vi "Server_L.vi"(8 "stop":bool, 9 "port":u16=13078, 10 "Wait(ms)":i32=500, 11 "Server Name":string="TCPService") -> ()   [LabVIEW 2012]
panel:
  out "error out":errorcluster
  in  "error in":errorcluster
  out "Host_IP":string
  out "Users":i32 caption="#Users"
  out "Active":bool
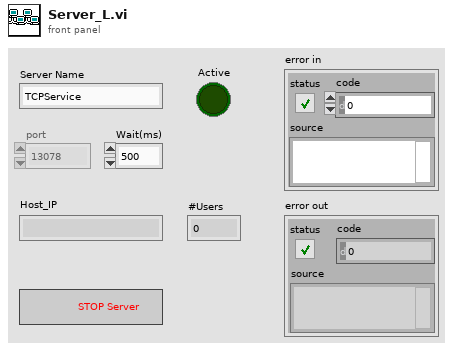
[diagram p1: front panel]
types:
  T1 = cluster{"rem addr":string, "conn ID":refnum<k5>}[]
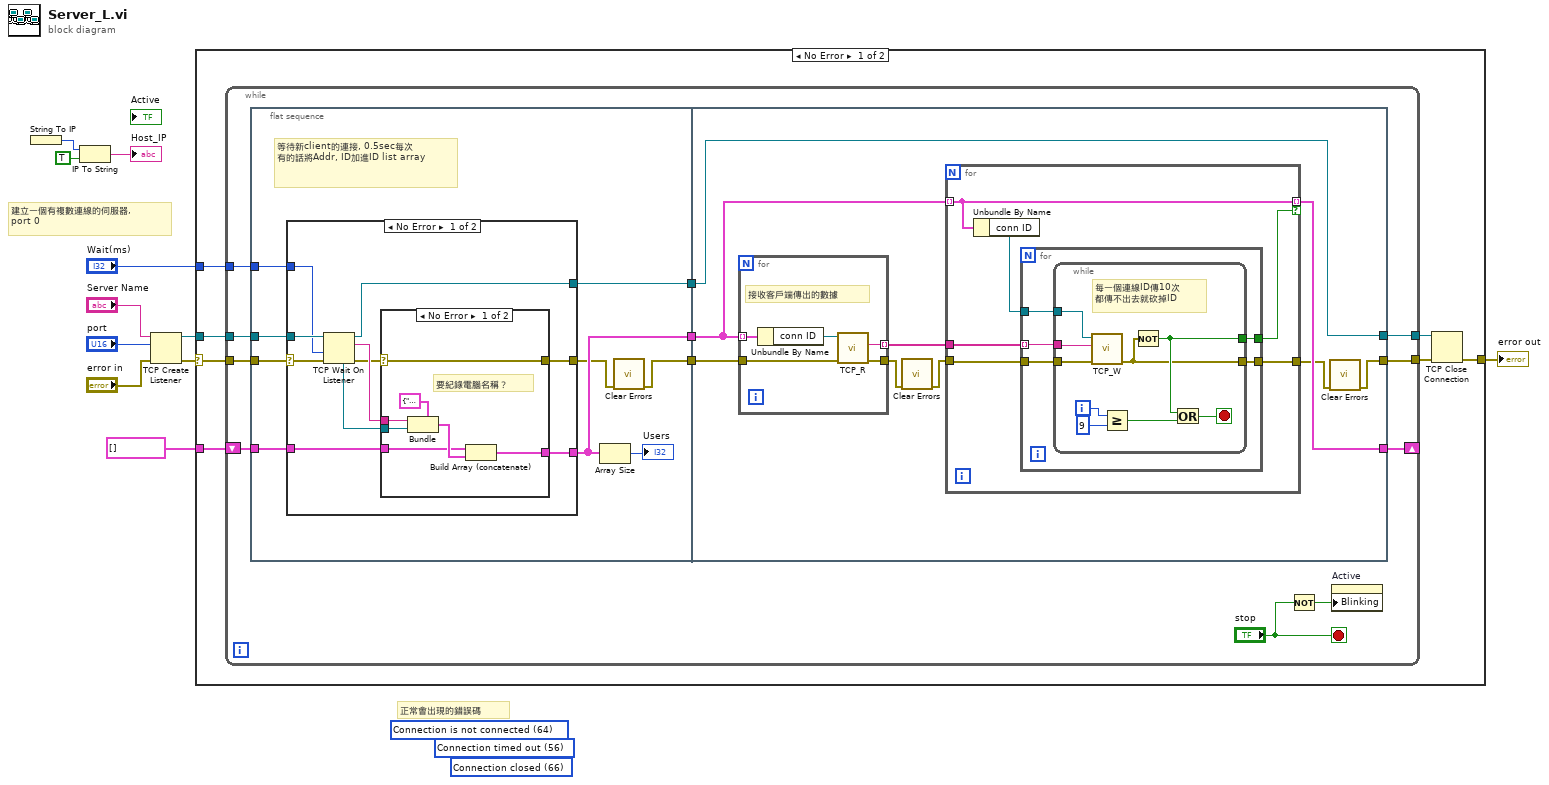
[diagram p0: block diagram]
diagram:
  (unwired) 56 items=["No Error", "Argument Error", "Memory Full", "Out of Zone", "End of File", "File Already Open", "Generic File IO Error", "File Not Found", "File Permission Error", "Disk Full", "Duplicate Path", "Too Many Files Open", "Not Enabled", "Resource File Not Found", "Cannot Add Resource", "Resource Not Found", "Image Not Found", "Image Memory Error", "Pen Does Not Exist", "Config Bad Type", "Config Token Not Found", "Config Parse Error", "Config Memory Error", "Bad External Code Format", "Bad External Code Offset", "External Code Not Present", "Null Window", "Destroy Window Mixup", "Null Menu", "Print Aborted", "Bad Print Record", "Print Driver Error", "Windows Error During Print", "Memory Error During Print", "Print Dialog Error", "Generic Print Error", "Invalid Device Refnum", "Device Not Found", "Device Parameter Error", "Device Unit Error", "Can't Open Device", "Device Call Aborted", "Generic Error", "Cancelled By User", "Object ID Too Low", "Object ID Too High", "Object Not In Heap", "Unknown Heap", "Bad DefProc ID", "DefProc Not In Table", "Message Out Of Range", "Null Method", "Unknown Message", "Manager Call Not Supported", "Bad address", "Connection In progress", "Connection timed out", "Connection is already in progress", "Network attribute not supported", "Network error", "Address in use", "System out of memory", "Connection aborted", "Connection refused", "Connection is not connected", "Connection is already connected", "Connection closed", "Initialize error (interapplication manager)", "Bad occurrence", "Wait on unbound occurrence handler", "Occurrence queue overflow", "Bad path", "Semaphore not signaled", "Unrecognized type (interapplication manager)"] ("2nd Error to Convert")
  (unwired) 66 items=["No Error", "Argument Error", "Memory Full", "Out of Zone", "End of File", "File Already Open", "Generic File IO Error", "File Not Found", "File Permission Error", "Disk Full", "Duplicate Path", "Too Many Files Open", "Not Enabled", "Resource File Not Found", "Cannot Add Resource", "Resource Not Found", "Image Not Found", "Image Memory Error", "Pen Does Not Exist", "Config Bad Type", "Config Token Not Found", "Config Parse Error", "Config Memory Error", "Bad External Code Format", "Bad External Code Offset", "External Code Not Present", "Null Window", "Destroy Window Mixup", "Null Menu", "Print Aborted", "Bad Print Record", "Print Driver Error", "Windows Error During Print", "Memory Error During Print", "Print Dialog Error", "Generic Print Error", "Invalid Device Refnum", "Device Not Found", "Device Parameter Error", "Device Unit Error", "Can't Open Device", "Device Call Aborted", "Generic Error", "Cancelled By User", "Object ID Too Low", "Object ID Too High", "Object Not In Heap", "Unknown Heap", "Bad DefProc ID", "DefProc Not In Table", "Message Out Of Range", "Null Method", "Unknown Message", "Manager Call Not Supported", "Bad address", "Connection In progress", "Connection timed out", "Connection is already in progress", "Network attribute not supported", "Network error", "Address in use", "System out of memory", "Connection aborted", "Connection refused", "Connection is not connected", "Connection is already connected", "Connection closed", "Initialize error (interapplication manager)", "Bad occurrence", "Wait on unbound occurrence handler", "Occurrence queue overflow", "Bad path", "Semaphore not signaled", "Unrecognized type (interapplication manager)"] ("3rd Error to Convert")
  (unwired) 64 items=["No Error", "Argument Error", "Memory Full", "Out of Zone", "End of File", "File Already Open", "Generic File IO Error", "File Not Found", "File Permission Error", "Disk Full", "Duplicate Path", "Too Many Files Open", "Not Enabled", "Resource File Not Found", "Cannot Add Resource", "Resource Not Found", "Image Not Found", "Image Memory Error", "Pen Does Not Exist", "Config Bad Type", "Config Token Not Found", "Config Parse Error", "Config Memory Error", "Bad External Code Format", "Bad External Code Offset", "External Code Not Present", "Null Window", "Destroy Window Mixup", "Null Menu", "Print Aborted", "Bad Print Record", "Print Driver Error", "Windows Error During Print", "Memory Error During Print", "Print Dialog Error", "Generic Print Error", "Invalid Device Refnum", "Device Not Found", "Device Parameter Error", "Device Unit Error", "Can't Open Device", "Device Call Aborted", "Generic Error", "Cancelled By User", "Object ID Too Low", "Object ID Too High", "Object Not In Heap", "Unknown Heap", "Bad DefProc ID", "DefProc Not In Table", "Message Out Of Range", "Null Method", "Unknown Message", "Manager Call Not Supported", "Bad address", "Connection In progress", "Connection timed out", "Connection is already in progress", "Network attribute not supported", "Network error", "Address in use", "System out of memory", "Connection aborted", "Connection refused", "Connection is not connected", "Connection is already connected", "Connection closed", "Initialize error (interapplication manager)", "Bad occurrence", "Wait on unbound occurrence handler", "Occurrence queue overflow", "Bad path", "Semaphore not signaled", "Unrecognized type (interapplication manager)"] ("1st Error to Convert")
  # "正常會出現的錯誤碼"
  # "建立一個有複數連線的伺服器,\nport 0"
  n1 = String To IP() -> (0:w8:u32)  [unwired: 1 in]
  n2 = IP To String(1:TRUE ("dot notation? (F)"), 2:w8) -> (0:→"Host_IP":string)
  n3 = TCP Create Listener(8:"error in", 10:"port", 11:"Server Name") -> (0:w10:errorcluster, 3:w9:refnum<k5>)  [unwired: 2 in, 1 out]
  n4 = case shown="No Error" w10 {
    selector: w10 -> [w16 w95]
    tunnel: w9 -> [w18 _]
    tunnel: T1 [] ("array") -> [w17 _]
    tunnel: [w12 w95] -> w2
    tunnel: "Wait(ms)" -> [w13 _]
    frame No Error {
      n5 = while {
        shift-right: [w27] -> _
        shift-left: w17 -> [w29]
        tunnel: w16 -> [w30]
        tunnel: w18 -> [w28]
        tunnel: [w24] -> w14
        tunnel: [w23] -> w15
        tunnel: w13 -> [w19]
        stop <- "stop" stop-if-true
        n6 = flat-sequence {
          tunnel: w30 -> [w38]
          tunnel: w29 -> [w39]
          tunnel: w28 -> [w37]
          tunnel: [w32] -> w22
          tunnel: [w35] -> w21
          tunnel: [w33] -> w20
          tunnel: w19 -> [w31]
          tunnel: [w68] -> w27
          tunnel: [w62] -> w24
          tunnel: [w61] -> w23
          tunnel: w22 -> [w61]
          tunnel: w21 -> [w67]
          tunnel: w20 -> [w63]
          frame #0 {
            # "等待新client的連接, 0.5sec每次\n有的話將Addr, ID加進ID list array"
            n7 = case shown="No Error" w38 {
              selector: w38 -> [w48 w60]
              tunnel: w37 -> [w49 _]
              tunnel: [w41 w60] -> w34
              tunnel: [w47 _] -> w32
              tunnel: [w46 w59] -> w35
              tunnel: w39 -> [w45 w59]
              tunnel: w31 -> [w40 _]
              frame No Error {
                n8 = TCP Wait On Listener(8:w48, 9:w40, 11:w49) -> (0:w42:errorcluster, 2:w43:string, 3:w47:refnum<k5>, 4:w44:refnum<k5>)  [unwired: 1 in, 1 out]
                n9 = case shown="No Error" w42 {
                  selector: w42 -> [w50 w57]
                  tunnel: [w56 w58] -> w46
                  tunnel: w45 -> [w54 w58]
                  tunnel: w44 -> [w51 _]
                  tunnel: w43 -> [w53 _]
                  tunnel: [w50 w57] -> w41
                  frame No Error {
                    # "要紀錄電腦名稱？"
                    n10 = Bundle(cluster=cluster{"rem addr":string, "conn ID":refnum<k5>} {"rem addr"="", "conn ID"=refnum}, "rem addr"=w53, "conn ID"=w51) -> (w55:cluster{"rem addr":string, "conn ID":refnum<k5>})
                    n11 = Build Array (concatenate)(w54, w55) -> (w56:T1)
                  }
                  frame Error {
                  }
                }
              }
              frame Error {
              }
            }
            n12 = Array Size(array=w35) -> (size(s)=→"Users":i32)
            n13 = call <vilib>:"Clear Errors.vi"("error in (no error)"=w34) -> ("error out"=w33:errorcluster)  [unwired: 6 in]
          }
          frame #1 {
            n14 = for {
              tunnel: w67 -> [w94] mode=indexing
              tunnel: [w91] -> w69 mode=indexing
              tunnel: [w92] -> w66
              tunnel: w63 -> [w90]
              # "接收客戶端傳出的數據"
              n15 = Unbundle By Name(w94) -> ("conn ID"=w93:refnum<k5>)
              n16 = call "TCP_R.vi"("error in"=w90, "connection ID"=w93) -> ("error out"=w92:errorcluster, "data out"=w91:string)  [unwired: 7 in, 1 out]
            }
            n17 = call <vilib>:"Clear Errors.vi"("error in (no error)"=w66) -> ("error out"=w65:errorcluster)  [unwired: 6 in]
            n18 = for {
              tunnel: w69 -> [w74]
              tunnel: w67 -> [w73] mode=indexing
              tunnel: [w73] -> w68 mode=indexing if=w72
              tunnel: w65 -> [w71]
              tunnel: [w70] -> w64
              n19 = Unbundle By Name(w73) -> ("conn ID"=w75:refnum<k5>)
              n20 = for {
                tunnel: w75 -> [w80]
                tunnel: w74 -> [w79] mode=indexing
                tunnel: [w78] -> w72
                tunnel: w71 -> [w77]
                tunnel: [w76] -> w70
                n21 = while {
                  tunnel: w80 -> [w85]
                  tunnel: w79 -> [w86]
                  tunnel: [w87] -> w78
                  tunnel: w77 -> [w84]
                  tunnel: [w83] -> w76
                  i -> [w82]
                  stop <- w89 stop-if-true
                  # "每一個連線ID傳10次\n都傳不出去就砍掉ID"
                  n22 = call "TCP_W.vi"("error in"=w84, "data in"=w86, "connection ID"=w85) -> ("error IO"=w83:errorcluster)  [unwired: 7 in, 1 out]
                  n23 = Greater Or Equal?(x=w82, y=9 ("x")) -> (x >= y?=w88:bool)
                  n24 = Not(x=w83) -> (.not. x?=w87:bool)
                  n25 = Or(x=w87, y=w88) -> (x .or. y?=w89:bool)
                }
              }
            }
            n26 = call <vilib>:"Clear Errors.vi"("error in (no error)"=w64) -> ("error out"=w62:errorcluster)  [unwired: 6 in]
          }
        }
        n27 = Not(x="stop") -> (.not. x?=w26:bool)
        n28 = property on="Active" class="Bool (strict)"("Blinking"=w26) -> ()  [unwired: 2 in, 2 out]
      }
      n29 = TCP Close Connection(connection ID=w15, error in (no error)=w14) -> (error out=w12:errorcluster)  [unwired: 1 in, 1 out]
    }
    frame Error {
    }
  }
  "error out" <- w2
